vi "Intial_N6705B_001.vi"(8 "error in (no error)":errorcluster {"code" format="%.0x"}, 10 "Channel Name (1) in":string="1", 11 "VISA Refnum in":refnum<visa-resource-name>="VAL_N6705B") -> (0 "error out":errorcluster, 2 "Channel Name (1) out":string, 3 "VISA Refnum out":refnum<visa-resource-name>)   [LabVIEW 2015]
uses:
  <instrlib>/Agilent N6700 Series/Agilent N6700 Series.lvlib
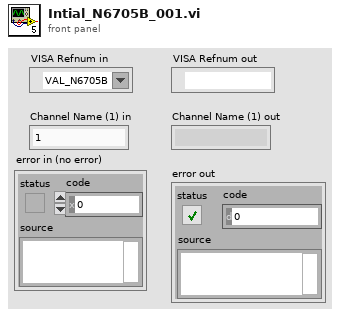
[diagram p1: front panel]
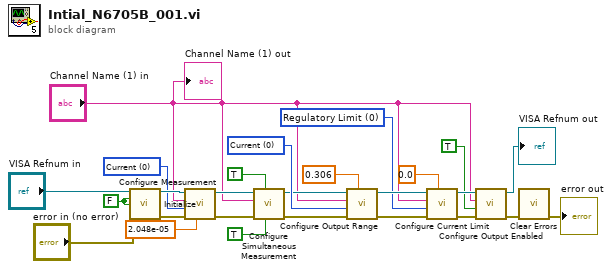
[diagram p0: block diagram]
diagram:
  w12 = 0 items=["Regulatory Limit", "Trip Limit"] ("Behavior (0: Regulatory Limit)")
  w17 = 0 items=["Voltage"=1, "Current"=0] ("Range Type (1: Voltage)")
  w19 = 0 items=["Voltage"=1, "Current"=0] ("Measurement Type (1: Voltage)")
  w18 = FALSE ("Reset? (T: Yes)")
  n1 = call <instrlib>:"Initialize.vi"("VISA resource name"="VISA Refnum in", "ID Query? (T: Yes)"=w18, "Reset? (T: Yes)"=w18, "error in (no error)"="error in (no error)") -> ("VISA resource name out"=w20:refnum<visa-resource-name>, "error out"=w21:errorcluster)  [unwired: 10 in]
  n2 = call <instrlib>:"Configure Measurement.vi"("Sample Interval (20.48e-6)"=2.048e-05, "error in (no error)"=w21, "Measurement Type (1: Voltage)"=w19, "Channel Name (1)"="Channel Name (1) in", "VISA resource name"=w20) -> ("error out"=w23:errorcluster, "VISA resource name out"=w22:refnum<visa-resource-name>)  [unwired: 5 in]
  n3 = call <instrlib>:"Configure Simultaneous Measurement.vi"("Enable Voltage Measurement (False)"=TRUE, "Enable Current Measurement (False)"=TRUE, "error in (no error)"=w23, "Channel Name (1)"="Channel Name (1) in", "VISA resource name"=w22) -> ("error out"=w14:errorcluster, "VISA resource name out"=w15:refnum<visa-resource-name>)  [unwired: 5 in]
  n4 = call <instrlib>:"Configure Output Range.vi"("Range (0.0)"=0.306, "error in (no error)"=w14, "Range Type (1: Voltage)"=w17, "Channel Name (1)"="Channel Name (1) in", "VISA resource name"=w15) -> ("error out"=w8:errorcluster, "VISA resource name out"=w13:refnum<visa-resource-name>)  [unwired: 5 in]
  n5 = call <instrlib>:"Configure Current Limit.vi"("Limit (0.0 amps)"=0.0, "error in (no error)"=w8, "Behavior (0: Regulatory Limit)"=w12, "Channel Name (1)"="Channel Name (1) in", "VISA resource name"=w13) -> ("error out"=w5:errorcluster, "VISA resource name out"=w10:refnum<visa-resource-name>)  [unwired: 5 in]
  n6 = call <instrlib>:"Configure Output Enabled.vi"("error in (no error)"=w5, "Enable Output (False)"=TRUE, "Channel Name (1)"="Channel Name (1) in", "VISA resource name"=w10) -> ("error out"=w4:errorcluster, "VISA resource name out"=→"VISA Refnum out":refnum<visa-resource-name>)  [unwired: 6 in]
  n7 = call <vilib>:"Clear Errors.vi"("error in (no error)"=w4) -> ("error out"=→"error out":errorcluster)  [unwired: 5 in, 1 out]
  "Channel Name (1) out" <- "Channel Name (1) in"
